vi "Main.vi"(11 "Module Admin":refnum<class "Delacor_lib_QMH_Module Admin.lvclass">) -> ()   [LabVIEW 2019, in "Calculadora.lvlib"]
doc: "This template is based off of the Queued Message Handler design pattern and the Queued Message Handler project template that ships with LabVIEW.\n\nThe main difference is that the queue is private to this module and communication between modules is performed via Broadcast and Request events.\n\nRequest events are wrapped in public API methods and are handled in the Event Handling Loop (EHL) of this VI. Any module can register for Broadcast events sent by this module. The EHL generates messages based on user interface actions.\n\nThe Message Handling Loop (MHL) processes messages generated by the EHL, or by other messages. The messages are string values, so new messages can be added easily to the Message Cases case structure in the MHL. Each message cluster can also provide an optional value for Message Data, which is a variant that can be converted to whatever message-specific data is required.\n_____\nBased on DQMH Project Template 6.1.0.94."
uses:
  Calculadora.lvlib
  <vilib>/Delacor/Delacor QMH/Libraries/Module Admin_class/Delacor_lib_QMH_Module Admin.lvclass
  Module Data--cluster.ctl
  Do Something Argument--cluster.ctl
  <vilib>/Delacor/Delacor QMH/Libraries/Message Queue_class/Delacor_lib_QMH_Message Queue.lvclass/Delacor_lib_QMH_Message Queue.ctl
  Do Something Else Argument--cluster.ctl
  Do Something Else and Wait for Reply Argument--cluster.ctl
  Do Something Else and Wait (Reply Payload)--cluster.ctl
  Stop Argument--cluster.ctl
  <vilib>/Delacor/Delacor QMH/Libraries/Module Admin_class/Delacor_lib_QMH_Module Admin.lvclass/Delacor_lib_QMH_Module Admin.ctl
  Suma Argument--cluster.ctl
  Resta Argument--cluster.ctl
  Multiplicacion Argument--cluster.ctl
  Division Argument--cluster.ctl
  Borrar Argument--cluster.ctl
  <vilib>/Utility/miscctls.llb/LVPointTypeDef.ctl
  <vilib>/Delacor/Delacor QMH/Libraries/Message Queue_class/Delacor_lib_QMH_Enqueue Message (Single).vi
  <vilib>/Delacor/Delacor QMH/Libraries/Module Admin_class/Delacor_lib_QMH_Get External Launch.vi
  <vilib>/Utility/error.llb/Error Cluster From Error Code.vi
  <vilib>/ErrorRing/Error Ring.xnode
  <vilib>/Delacor/Delacor QMH/Libraries/Message Queue_class/Delacor_lib_QMH_Message Queue.lvclass
panel:
  out "error out":errorcluster
  out "X":dbl
  out "Status":string
  in  "Simulate MHL Error":bool
  in  "Simulate EHL Error":bool
  in  "Do Something Else <Replace Me>":bool
  in  "Do Something <Replace Me>":bool
  # "These controls have associated \"Value Changed\" events configured in the Event Structure on the diagram.\n\nReplace them (and reconfigure the Event Structure) with the controls you need for your application. \n\nOther QMH Modules communicate with this Module via its Public API (wrappers for its Request Events).\n\nThis Module communicates with other Modules via its Broadcast Events.\nAny module that wants to get these messages, just registers for this module's Broadcast events."
  # "This template is for the Delacor Modified Queued Message Handler design pattern.\n\nSee the block diagram for more information on how to use this template."
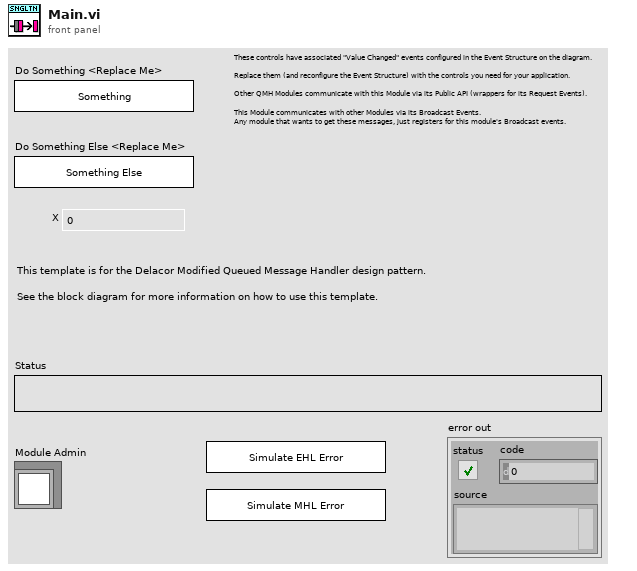
[diagram p1: front panel]
types:
  T1 = typedef "Calculadora.lvlib/Request Events--cluster.ctl" = cluster{"Stop Module":refnum<user-event>, "Do Something":refnum<user-event>, "Do Something Else":refnum<user-event>, "Do Something Else and Wait for Reply":refnum<user-event>, "Show Panel":refnum<user-event>, "Hide Panel":refnum<user-event>, "Get Module Execution Status":refnum<user-event>, "Show Diagram":refnum<user-event>, "Suma":refnum<user-event>, "Resta":refnum<user-event>, "Multiplicacion":refnum<user-event>, "Division":refnum<user-event>, "Borrar":refnum<user-event>}
  T2 = typedef "Calculadora.lvlib/Module Data--cluster.ctl" = cluster{"Status":string, "Resultado":dbl}
  T3 = typedef "Calculadora.lvlib/Do Something Argument--cluster.ctl" = cluster{"Do Something Msg":string}
  T4 = typedef "Calculadora.lvlib/Do Something Else Argument--cluster.ctl" = cluster{"Do Something Else Msg":string, "X":dbl}
  T5 = typedef "Calculadora.lvlib/Do Something Else and Wait for Reply Argument--cluster.ctl" = cluster{"Do Something Else Msg":string, "X":dbl, "Wait Notifier":refnum<notifier>, "wait for reply":bool}
  T6 = enum32{"invalid lock state", "Not Locked", "Locked (No Password)", "Password-protected"}
  T7 = typedef "Calculadora.lvlib/Stop Argument--cluster.ctl" = cluster{"Origin":string, "Exit via Stop Module Req?":bool, "Wait for Module to stop?":bool}
  T8 = typedef "Calculadora.lvlib/Suma Argument--cluster.ctl" = cluster{"Numero":dbl}
  T9 = typedef "Calculadora.lvlib/Resta Argument--cluster.ctl" = cluster{"Numero":dbl}
  T10 = typedef "Calculadora.lvlib/Multiplicacion Argument--cluster.ctl" = cluster{"Numero":dbl}
  T11 = typedef "Calculadora.lvlib/Division Argument--cluster.ctl" = cluster{"Numero":dbl}
  T12 = typedef "Calculadora.lvlib/Borrar Argument--cluster.ctl" = cluster{"Boolean":bool}
  T13 = typedef "LVPointTypeDef.ctl" = cluster{"Horizontal":i16, "Vertical":i16}
  T14 = enum32{"Invalid", "Standard", "Closed", "Hidden", "Minimized", "Maximized"}
  T15 = typedef "Calculadora.lvlib/Do Something Else and Wait (Reply Payload)--cluster.ctl" = cluster{"Value":dbl, "error":errorcluster}
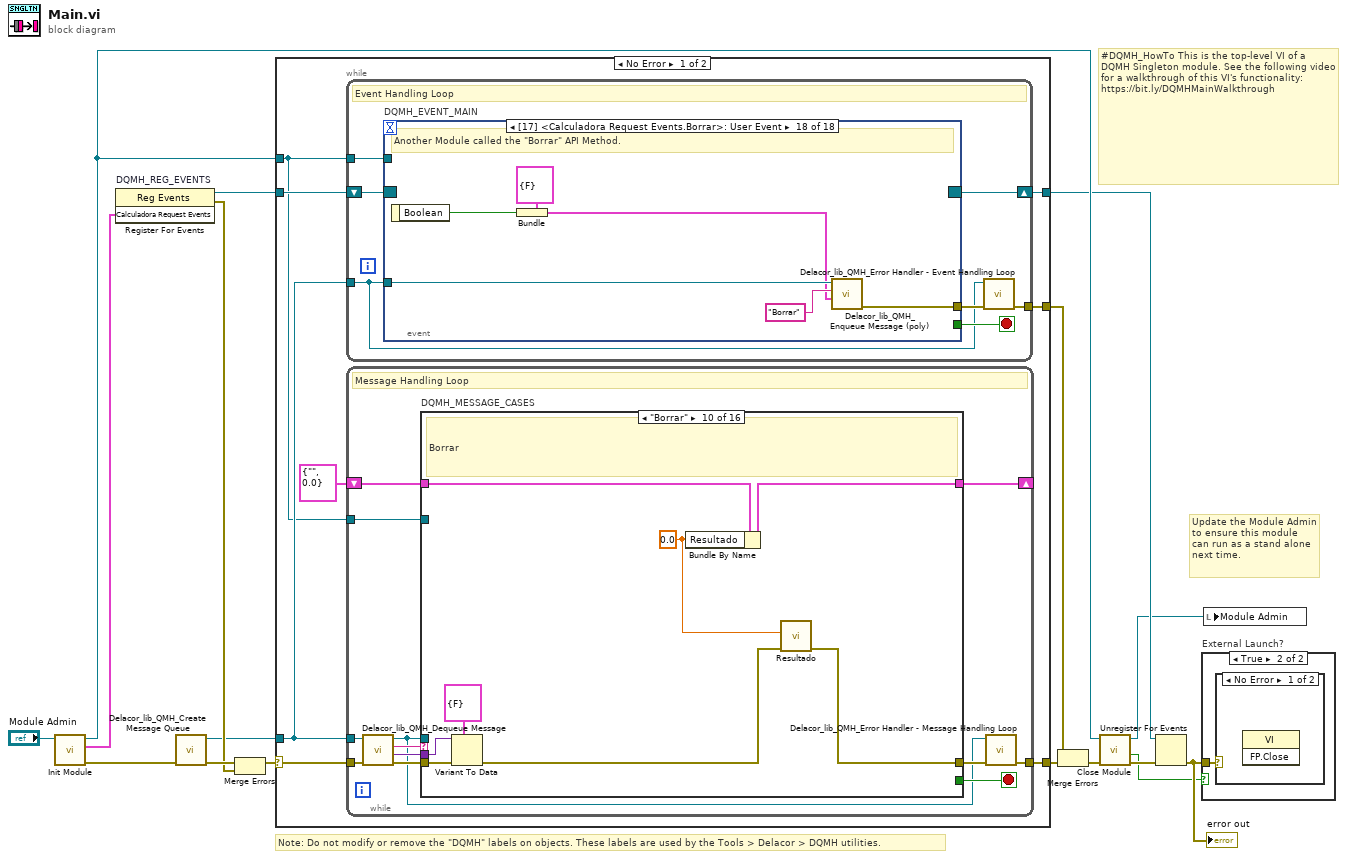
[diagram p0: block diagram]
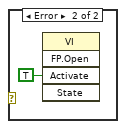
[diagram p3: hidden frame]
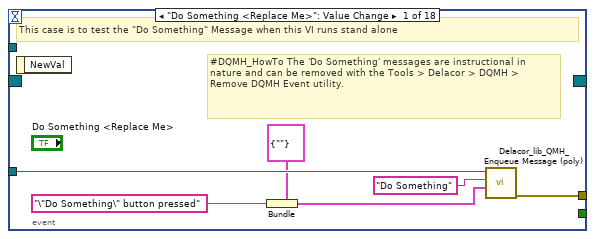
[diagram p4: hidden frame]
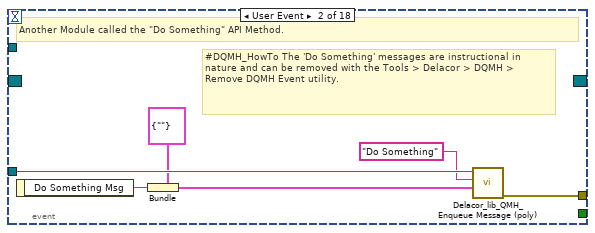
[diagram p5: hidden frame]
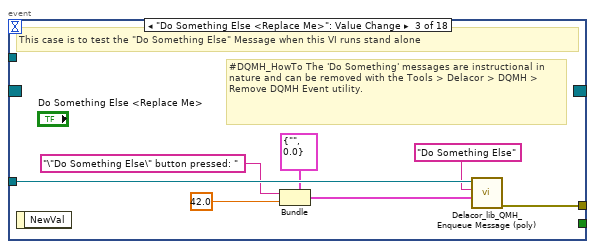
[diagram p6: hidden frame]
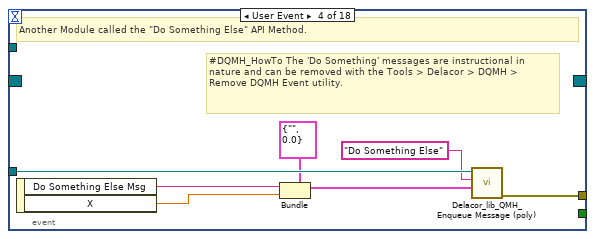
[diagram p7: hidden frame]
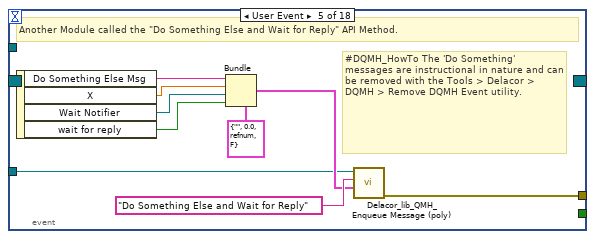
[diagram p8: hidden frame]
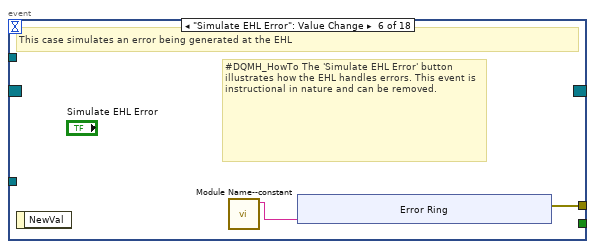
[diagram p9: hidden frame]
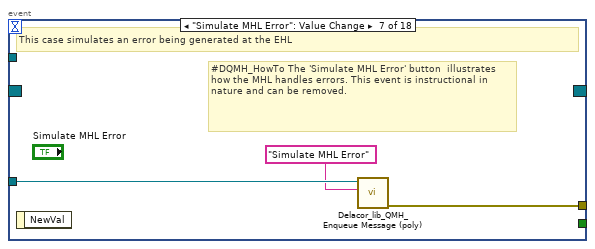
[diagram p10: hidden frame]
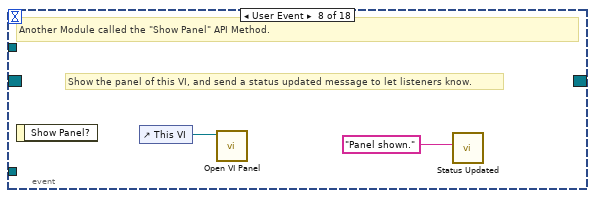
[diagram p11: hidden frame]
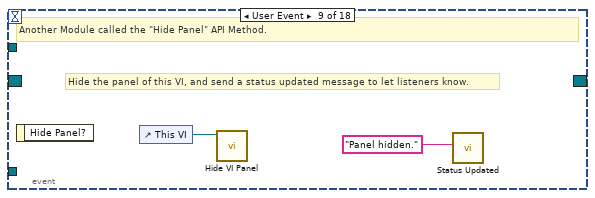
[diagram p12: hidden frame]
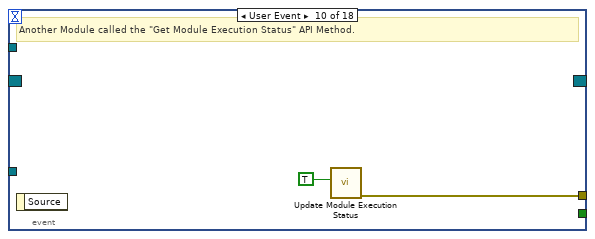
[diagram p13: hidden frame]
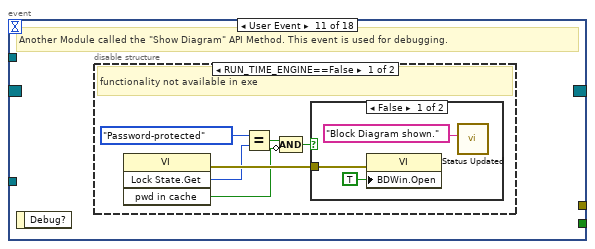
[diagram p14: hidden frame]
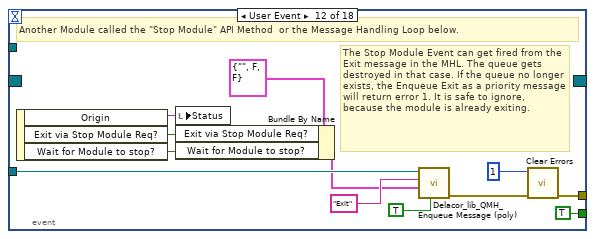
[diagram p17: hidden frame]
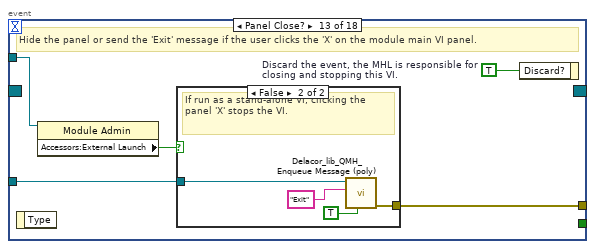
[diagram p18: hidden frame]
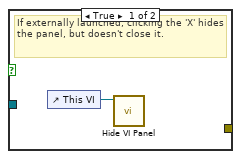
[diagram p19: hidden frame]
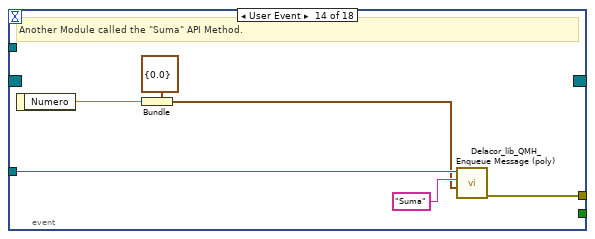
[diagram p20: hidden frame]
diagram:
  # "#DQMH_HowTo This is the top-level VI of a DQMH Singleton module. See the following video for a walkthrough of this VI's functionality: https://bit.ly/DQMHMainWalkthrough"
  # "Note: Do not modify or remove the \"DQMH\" labels on objects. These labels are used by the Tools > Delacor > DQMH utilities."
  # "Update the Module Admin to ensure this module can run as a stand alone next time."
  n1 = call "Init Module.vi"("Singleton Module Admin in"="Module Admin") -> ("error out"=w16:errorcluster, "Calculadora Request Events"=w5:T1, "Singleton Module Admin out"=w8:refnum<class "Delacor_lib_QMH_Module Admin.lvclass">)  [unwired: 8 in]
  n2 = register-events "DQMH_REG_EVENTS"(w5) -> (reference out=w6:refnum<event-registration>, error out=w9:errorcluster)  [unwired: 2 in]
  n3 = call <vilib>:"Delacor_lib_QMH_Create Message Queue.vi"("error in"=w16) -> ("error out"=w11:errorcluster, "Message Queue"=w4:refnum<class "Delacor_lib_QMH_Message Queue.lvclass">)  [unwired: 9 in]
  n4 = Merge Errors(w11, w9) -> (w10:errorcluster)
  n5 = case shown="No Error" w10 {
    selector: w10 -> [w23 w345]
    tunnel: [w25 w344] -> w17
    tunnel: [w22 w350] -> w7
    tunnel: w6 -> [w20 w350]
    tunnel: w4 -> [w19 w343]
    tunnel: [w24 _] -> w14
    tunnel: w8 -> [w18 w346]
    frame No Error {
      n6 = while {
        tunnel: w19 -> [w26]
        shift-right: [w29] -> w22
        shift-left: w20 -> [w30]
        tunnel: [w31] -> w24
        tunnel: w18 -> [w27]
        stop <- w28 stop-if-true
        # "Event Handling Loop"
        n7 = event "DQMH_EVENT_MAIN" shown="[17] <Calculadora Request Events.Borrar>: User Event" {
          selector: w30 -> [_ _ _ _ _ _ _ _ _ _ _ _ _ _ _ _ _ _]
          dyn-events: [_ _ _ _ _ _ _ _ _ _ _ _ _ _ _ _ _ _] -> w29
          timeout: _ -> [_ _ _ _ _ _ _ _ _ _ _ _ _ _ _ _ _ _]
          tunnel: [_ _ _ _ _ _ _ _ _ _ _ TRUE ("Discard?") _ _ _ _ _ _] -> w28
          tunnel: w26 -> [w37 w43 w50 w57 w60 _ w78 _ _ _ _ w102 w109 w122 w128 w134 w140 w146]
          tunnel: [w38 w44 w51 w58 w67 w69 w79 _ _ w85 _ w105 w111 w117 w123 w129 w135 w141] -> w32
          tunnel: w27 -> [_ _ _ _ _ _ _ _ _ _ _ _ w108 _ _ _ _ _]
          event "Do Something <Replace Me>": Value Change {
            # "#DQMH_HowTo The 'Do Something' messages are instructional in nature and can be removed with the Tools > Delacor > DQMH > Remove DQMH Event utility."
            # "This case is to test the \"Do Something\" Message when this VI runs stand alone"
            n8 = event-data() -> ()  [unwired: 1 in, 1 out]
            n9 = Bundle(cluster=T3 {"Do Something Msg"=""} ("Do Something Argument"), "Do Something Msg"="\"Do Something\" button pressed" ("\"Do Something\" button pressed")) -> (w33:T3)
            n10 = call-poly <vilib>:"Delacor_lib_QMH_Enqueue Message (poly).vi"("Message Data"=w33, "Message"="Do Something", "Message Queue in"=w37) -> ("error out"=w38:errorcluster)  [unwired: 7 in, 1 out]
          }
          event User Event {
            # "#DQMH_HowTo The 'Do Something' messages are instructional in nature and can be removed with the Tools > Delacor > DQMH > Remove DQMH Event utility."
            # "Another Module called the \"Do Something\" API Method."
            n11 = event-data() -> ("Do Something Msg"=w40:string)  [unwired: 1 in]
            n12 = Bundle(cluster=T3 {"Do Something Msg"=""} ("Do Something Argument"), "Do Something Msg"=w40) -> (w39:T3)
            n13 = call-poly <vilib>:"Delacor_lib_QMH_Enqueue Message (poly).vi"("Message Data"=w39, "Message"="Do Something", "Message Queue in"=w43) -> ("error out"=w44:errorcluster)  [unwired: 7 in, 1 out]
          }
          event "Do Something Else <Replace Me>": Value Change {
            # "#DQMH_HowTo The 'Do Something' messages are instructional in nature and can be removed with the Tools > Delacor > DQMH > Remove DQMH Event utility."
            # "This case is to test the \"Do Something Else\" Message when this VI runs stand alone"
            n14 = event-data() -> ()  [unwired: 1 in, 1 out]
            n15 = Bundle(cluster=T4 {"Do Something Else Msg"="", "X"=0.0} ("Do Something Else Argument"), "Do Something Else Msg"="\"Do Something Else\" button pressed: " ("\"Do Something Else\" button pressed"), "X"=42.0) -> (w47:T4)
            n16 = call-poly <vilib>:"Delacor_lib_QMH_Enqueue Message (poly).vi"("Message Data"=w47, "Message"="Do Something Else", "Message Queue in"=w50) -> ("error out"=w51:errorcluster)  [unwired: 7 in, 1 out]
          }
          event User Event {
            # "#DQMH_HowTo The 'Do Something' messages are instructional in nature and can be removed with the Tools > Delacor > DQMH > Remove DQMH Event utility."
            # "Another Module called the \"Do Something Else\" API Method."
            n17 = event-data() -> ("Do Something Else Msg"=w53:string, "X"=w52:dbl)  [unwired: 1 in]
            n18 = Bundle(cluster=T4 {"Do Something Else Msg"="", "X"=0.0} ("Do Something Else Argument"), "Do Something Else Msg"=w53, "X"=w52) -> (w54:T4)
            n19 = call-poly <vilib>:"Delacor_lib_QMH_Enqueue Message (poly).vi"("Message Data"=w54, "Message"="Do Something Else", "Message Queue in"=w57) -> ("error out"=w58:errorcluster)  [unwired: 7 in, 1 out]
          }
          event User Event {
            # "#DQMH_HowTo The 'Do Something' messages are instructional in nature and can be removed with the Tools > Delacor > DQMH > Remove DQMH Event utility."
            # "Another Module called the \"Do Something Else and Wait for Reply\" API Method."
            n20 = event-data() -> ("Do Something Else Msg"=w63:string, "X"=w62:dbl, "Wait Notifier"=w61:refnum<notifier>, "wait for reply"=w59:bool)  [unwired: 1 in]
            n21 = Bundle(cluster=T5 {"Do Something Else Msg"="", "X"=0.0, "Wait Notifier"=refnum, "wait for reply"=FALSE} ("Do Something Else and Wait for Reply Argument"), "Do Something Else Msg"=w63, "X"=w62, "Wait Notifier"=w61, "wait for reply"=w59) -> (w64:T5)
            n22 = call-poly <vilib>:"Delacor_lib_QMH_Enqueue Message (poly).vi"("Message Data"=w64, "Message"="Do Something Else and Wait for Reply", "Message Queue in"=w60) -> ("error out"=w67:errorcluster)  [unwired: 7 in, 1 out]
          }
          event "Simulate EHL Error": Value Change {
            # "#DQMH_HowTo The 'Simulate EHL Error' button  illustrates how the EHL handles errors. This event is instructional in nature and can be removed."
            # "This case simulates an error being generated at the EHL"
            n23 = event-data() -> ()  [unwired: 1 in, 1 out]
            n24 = call "Module Name--constant.vi"() -> ("Module Name"=w68:string)  [unwired: 11 in]
            n25 = xnode "Error Ring"("parameter 0"=w68) -> ("error out"=w69:errorcluster)
          }
          event "Simulate MHL Error": Value Change {
            # "#DQMH_HowTo The 'Simulate MHL Error' button  illustrates how the MHL handles errors. This event is instructional in nature and can be removed."
            # "This case simulates an error being generated at the EHL"
            n26 = event-data() -> ()  [unwired: 1 in, 1 out]
            n27 = call-poly <vilib>:"Delacor_lib_QMH_Enqueue Message (poly).vi"("Message"="Simulate MHL Error", "Message Queue in"=w78) -> ("error out"=w79:errorcluster)  [unwired: 8 in, 1 out]
          }
          event User Event {
            # "Show the panel of this VI, and send a status updated message to let listeners know."
            # "Another Module called the \"Show Panel\" API Method."
            n28 = event-data() -> ()  [unwired: 1 in, 1 out]
            n29 = control-ref of="This VI"() -> (w81:refnum<vi>)
            n30 = call "Open VI Panel.vi"("VI"=w81) -> ()  [unwired: 10 in, 1 out]
            n31 = call "Status Updated.vi"("Status"="Panel shown." ("format string")) -> ()  [unwired: 10 in, 1 out]
          }
          event User Event {
            # "Hide the panel of this VI, and send a status updated message to let listeners know."
            # "Another Module called the \"Hide Panel\" API Method."
            n32 = event-data() -> ()  [unwired: 1 in, 1 out]
            n33 = control-ref of="This VI"() -> (w83:refnum<vi>)
            n34 = call "Hide VI Panel.vi"("VI"=w83) -> ()  [unwired: 10 in, 1 out]
            n35 = call "Status Updated.vi"("Status"="Panel hidden." ("format string")) -> ()  [unwired: 10 in, 1 out]
          }
          event User Event {
            # "Another Module called the \"Get Module Execution Status\" API Method."
            n36 = event-data() -> ()  [unwired: 1 in, 1 out]
            n37 = call "Update Module Execution Status.vi"("Running?"=TRUE) -> ("error out"=w85:errorcluster)  [unwired: 10 in]
          }
          event User Event {
            # "Another Module called the \"Show Diagram\" API Method. This event is used for debugging."
            n38 = event-data() -> ()  [unwired: 1 in, 1 out]
            n39 = disable-structure shown="RUN_TIME_ENGINE==False" {
              frame condition #0 (active) {
                # "functionality not available in exe"
                n40 = invoke class="VI" method="Lock State.Get"() -> (error out=w91:errorcluster, "Get Lock State"=w90:T6, "pwd in cache"=w87:bool)  [unwired: 4 in, 1 out]
                n41 = Equal?(x=T6."Password-protected", y=w90) -> (x = y?=w88:bool)
                n42 = Compound Arithmetic op=AND(w88, invert w87) -> (w86:bool)
                n43 = case shown="False" w86 {
                  tunnel: w91 -> [w94 _]
                  frame False {
                    n44 = property class="VI"(error in=w94, "BDWin.Open"=TRUE ("Block Diagram Window:Open")) -> ()  [unwired: 1 in, 2 out]
                    n45 = call "Status Updated.vi"("Status"="Block Diagram shown." ("format string")) -> ()  [unwired: 10 in, 1 out]
                  }
                  frame True {
                    # "Password-protected VI, and the password is not in the cache. Do not show the diagram."
                  }
                }
              }
              frame condition #1 {
              }
            }
          }
          event User Event {
            # "The Stop Module Event can get fired from the Exit message in the MHL. The queue gets destroyed in that case. If the queue no longer exists, the Enqueue Exit as a priority message will return error 1. It is safe to ignore, because the module is already exiting."
            # "Another Module called the \"Stop Module\" API Method  or the Message Handling Loop below."
            n46 = event-data() -> ("Origin"=w101:string, "Exit via Stop Module Req?"=w97:bool, "Wait for Module to stop?"=w96:bool)  [unwired: 1 in]
            n47 = local write "Status"(w101) -> ()
            n48 = Bundle By Name(cluster=T7 {"Origin"="", "Exit via Stop Module Req?"=FALSE, "Wait for Module to stop?"=FALSE} ("Stop Argument"), "Exit via Stop Module Req?"=w97, "Wait for Module to stop?"=w96) -> (w95:T7)
            n49 = call-poly <vilib>:"Delacor_lib_QMH_Enqueue Message (poly).vi"("Priority Message? (F)"=TRUE, "Message Data"=w95, "Message"="Exit", "Message Queue in"=w102) -> ("error out"=w106:errorcluster)  [unwired: 6 in, 1 out]
            n50 = call <vilib>:"Clear Errors.vi"("error in (no error)"=w106, "specific error code to clear (0: all)"=1) -> ("error out"=w105:errorcluster)  [unwired: 4 in, 1 out]
          }
          event Panel Close? {
            w110 = TRUE  # Discard the event, the MHL is responsible for closing and stopping this VI.
            # "Hide the panel or send the 'Exit' message if the user clicks the 'X' on the module main VI panel."
            n51 = event-data() -> ()  [unwired: 1 in, 1 out]
            n52 = property class="Module Admin"(reference=w108) -> ("Accessors:External Launch"=w107:bool)  [unwired: 1 in, 2 out]
            n53 = case shown="False" w107 {
              tunnel: w109 -> [_ w115]
              tunnel: [_ w116] -> w111
              frame True {
                # "If externally launched, clicking the 'X' hides the panel, but doesn't close it."
                n54 = control-ref of="This VI"() -> (w112:refnum<vi>)
                n55 = call "Hide VI Panel.vi"("VI"=w112) -> ()  [unwired: 10 in, 1 out]
              }
              frame False {
                # "If run as a stand-alone VI, clicking the panel 'X' stops the VI."
                n56 = call-poly <vilib>:"Delacor_lib_QMH_Enqueue Message (poly).vi"("Priority Message? (F)"=TRUE, "Message"="Exit", "Message Queue in"=w115) -> ("error out"=w116:errorcluster)  [unwired: 7 in, 1 out]
              }
            }
            n57 = event-data("Discard?"=w110) -> ()  [unwired: 1 in, 1 out]
          }
          event User Event {
            # "Another Module called the \"Suma\" API Method."
            n58 = event-data() -> ("Numero"=w118:dbl)  [unwired: 1 in]
            n59 = Bundle(cluster=T8 {"Numero"=0.0} ("Suma Argument"), "Numero"=w118) -> (w119:T8)
            n60 = call-poly <vilib>:"Delacor_lib_QMH_Enqueue Message (poly).vi"("Message Data"=w119, "Message"="Suma", "Message Queue in"=w122) -> ("error out"=w117:errorcluster)  [unwired: 7 in, 1 out]
          }
          event User Event {
            # "Another Module called the \"Resta\" API Method."
            n61 = event-data() -> ("Numero"=w124:dbl)  [unwired: 1 in]
            n62 = Bundle(cluster=T9 {"Numero"=0.0} ("Resta Argument"), "Numero"=w124) -> (w125:T9)
            n63 = call-poly <vilib>:"Delacor_lib_QMH_Enqueue Message (poly).vi"("Message Data"=w125, "Message"="Resta", "Message Queue in"=w128) -> ("error out"=w123:errorcluster)  [unwired: 7 in, 1 out]
          }
          event User Event {
            # "Another Module called the \"Multiplicacion\" API Method."
            n64 = event-data() -> ("Numero"=w130:dbl)  [unwired: 1 in]
            n65 = Bundle(cluster=T10 {"Numero"=0.0} ("Multiplicacion Argument"), "Numero"=w130) -> (w131:T10)
            n66 = call-poly <vilib>:"Delacor_lib_QMH_Enqueue Message (poly).vi"("Message Data"=w131, "Message"="Multiplicacion", "Message Queue in"=w134) -> ("error out"=w129:errorcluster)  [unwired: 7 in, 1 out]
          }
          event User Event {
            # "Another Module called the \"Division\" API Method."
            n67 = event-data() -> ("Numero"=w136:dbl)  [unwired: 1 in]
            n68 = Bundle(cluster=T11 {"Numero"=0.0} ("Division Argument"), "Numero"=w136) -> (w137:T11)
            n69 = call-poly <vilib>:"Delacor_lib_QMH_Enqueue Message (poly).vi"("Message Data"=w137, "Message"="Division", "Message Queue in"=w140) -> ("error out"=w135:errorcluster)  [unwired: 7 in, 1 out]
          }
          event User Event {
            # "Another Module called the \"Borrar\" API Method."
            n70 = event-data() -> ("Boolean"=w142:bool)  [unwired: 1 in]
            n71 = Bundle(cluster=T12 {"Boolean"=FALSE} ("Borrar Argument"), "Boolean"=w142) -> (w143:T12)
            n72 = call-poly <vilib>:"Delacor_lib_QMH_Enqueue Message (poly).vi"("Message Data"=w143, "Message"="Borrar", "Message Queue in"=w146) -> ("error out"=w141:errorcluster)  [unwired: 7 in, 1 out]
          }
        }
        n73 = call-dynamic "Delacor_lib_QMH_Error Handler - Event Handling Loop.vi"("error in"=w32, "Message Queue in"=w26) -> ("dup error in"=w31:errorcluster)  [unwired: 8 in, 1 out]
      }
      n74 = while {
        tunnel: w19 -> [w149]
        shift-right: [w153] -> _
        shift-left: T2 {"Status"="", "Resultado"=0.0} ("Data Cluster") -> [w154]
        tunnel: w23 -> [w157]
        tunnel: [w155] -> w25
        tunnel: w18 -> [w147]
        stop <- w152 stop-if-true
        # "Message Handling Loop"
        n75 = call-dynamic "Delacor_lib_QMH_Dequeue Message.vi"("error in"=w157, "Message Queue in"=w149) -> ("error out"=w156:errorcluster, "Message Data"=w150:variant, "Message"=w151:string, "Message Queue out"=w148:refnum<class "Delacor_lib_QMH_Message Queue.lvclass">)  [unwired: 6 in]
        n76 = case "DQMH_MESSAGE_CASES" shown="\"Borrar\"" w151 {
          selector: w151 -> [_ _ _ _ _ _ _ _ _ _ _ _ _ _ _ w330]
          tunnel: w148 -> [_ _ _ _ _ _ _ _ _ _ _ _ _ w300 w322 _]
          tunnel: w156 -> [w177 w181 w189 w198 w217 w240 w250 w261 w272 w280 w283 w285 w290 w307 w328 w332]
          tunnel: [w175 w181 w187 w197 w216 w230 w249 w251 w262 w273 w282 w285 w289 w303 w325 w333] -> w158
          tunnel: w154 -> [w166 w180 w186 w196 w214 w236 w242 w254 w265 w279 w281 w284 w287 w302 w321 w331]
          tunnel: [w165 w180 w186 w196 w214 w233 w241 w253 w264 w276 w281 w284 w287 w302 w321 w331] -> w153
          tunnel: [_ _ _ _ _ _ _ _ _ _ _ _ _ _ w320 _] -> w152
          tunnel: w150 -> [_ _ w185 w193 w211 w239 w248 w260 w271 w278 _ _ _ w301 w319 _]
          tunnel: w147 -> [w167 _ _ _ _ _ _ _ _ _ _ _ _ w299 w314 _]
          frame "Initialize" {
            w161 = "Initial Message" ("Initial Message")
            # "Initialize - Any operation that needs to be done before the module can receive messages. Synchronize Caller Events.vi will inform Start Module.vi that the module has launched and is ready to receive messages. Module Did Init.vi will broadcast that the module initialized."
            n77 = call "Synchronize Caller Events.vi"("error in (no error)"=w177, "Singleton Module Admin in"=w167) -> ("error out"=w176:errorcluster, "Singleton Module Admin out"=w162:refnum<class "Delacor_lib_QMH_Module Admin.lvclass">)  [unwired: 8 in]
            n78 = property class="Module Admin"(reference=w162) -> ("Accessors:External Launch"=w171:bool)  [unwired: 1 in, 2 out]
            n79 = Select(t=T14."Hidden" ("State"), s=w171, f=T14."Standard" ("State")) -> (s? t:f=w168:T14)
            n80 = call "Module Name--constant.vi"() -> ("Module Name"=w174:string)  [unwired: 11 in]
            n81 = property class="VI"("Front Panel.Title"=w174) -> (reference out=w173:refnum<vi>, error out=w179:errorcluster)  [unwired: 2 in]
            n82 = call "Module Name--constant.vi"() -> ("Module Name"=w163:string)  [unwired: 11 in]
            n83 = invoke class="VI" method="FP.Open"(reference=w173, error in=w179, "State"=w168) -> (reference out=w172:refnum<vi>, error out=w178:errorcluster)  [unwired: 2 in, 3 out]
            n84 = Bundle By Name(cluster=w166, "Resultado"=0.0, "Status"=w161) -> (w165:T2)
            n85 = call "Module Did Init.vi"("error in (no error)"=w176, "Initialized?"=TRUE, "Origin"=w163) -> ("error out"=w175:errorcluster)  [unwired: 8 in]
            n86 = invoke class="VI" method="FP.Center"(reference=w172, error in=w178) -> ()  [unwired: 1 in, 3 out]
            n87 = property on="Pane" class="Pane"("Origin"=T13 {"Horizontal"=0, "Vertical"=0}) -> ()  [unwired: 2 in, 2 out]
            "Status" <- w161
          }
          frame "---Module Specific---" {
            # "Separator -- The following cases handle messages specific to this Module."
          }
          frame "Do Something" {
            # "#DQMH_HowTo The 'Do Something' messages are instructional in nature and can be removed with the Tools > Delacor > DQMH > Remove DQMH Event utility."
            # "Do Something - Replace this message with functionality for your own application. Note that this message also fires the \"Did Something\" broadcast event."
            n88 = Variant To Data(error in=w189, type=T3 {"Do Something Msg"=""} ("Do Something Argument"), Variant=w185) -> (data=w184:T3, error out=w188:errorcluster)
            n89 = Unbundle By Name(w184) -> ("Do Something Msg"=w182:string)
            n90 = call "Did Something.vi"("error in (no error)"=w188, "Did Something Msg"=w182) -> ("error out"=w187:errorcluster)  [unwired: 9 in]
            n91 = local write "Status"(w182) -> ()
            n92 = call "Status Updated.vi"("Status"=w182) -> ()  [unwired: 10 in, 1 out]
          }
          frame "Do Something Else" {
            # "#DQMH_HowTo The 'Do Something' messages are instructional in nature and can be removed with the Tools > Delacor > DQMH > Remove DQMH Event utility."
            # "Do Something Else - Replace this message with functionality for your own application."
            n93 = Variant To Data(error in=w198, type=T4 {"Do Something Else Msg"="", "X"=0.0} ("Do Something Else Argument"), Variant=w193) -> (data=w194:T4, error out=w197:errorcluster)
            n94 = Unbundle By Name(w194) -> ("Do Something Else Msg"=w192:string, "X"=w191:dbl)
            "X" <- w191
            n95 = Format Into String(initial string=w192, w191) -> (resulting string=w190:string)  [unwired: 2 in, 1 out]
            n96 = local write "Status"(w190) -> ()
            n97 = call "Status Updated.vi"("Status"=w190) -> ()  [unwired: 10 in, 1 out]
          }
          frame "Do Something Else and Wait for Reply" {
            w206 = "X(%.2f)+Offset(%.2f)=%.2f"  # status message format string
            # "#DQMH_HowTo The 'Do Something' messages are instructional in nature and can be removed."
            # "Send back X with a random offset"
            # "Do Something Else and Wait for Reply - Replace this message with functionality for your own application. Note that this message must fire a notifier to let callers know it has finished execution, and it returns an error if the 'Value' is negative."
            n98 = Random Number (0-1)() -> (number: 0 to 1=w208:dbl)
            n99 = Variant To Data(error in=w217, type=T5 {"Do Something Else Msg"="", "X"=0.0, "Wait Notifier"=refnum, "wait for reply"=FALSE} ("Do Something Else and Wait for Reply Argument"), Variant=w211) -> (data=w212:T5, error out=w215:errorcluster)
            n100 = Unbundle By Name(w212) -> ("Wait Notifier"=w199:refnum<notifier>, "Do Something Else Msg"=w210:string, "X"=w207:dbl, "wait for reply"=w203:bool)
            n101 = Add(x=w208, y=w207) -> (x+y=w202:dbl)
            n102 = local write "X"(w207) -> ()
            n103 = Less Than 0?(x=w202) -> (x < 0?=w205:bool)
            n104 = Format Into String(format string=w206, initial string=w210, w207, w208, w202) -> (resulting string=w204:string)  [unwired: 1 in, 1 out]
            n105 = case shown="True" w205 {
              tunnel: [_ w224] -> w200
              frame False {
              }
              frame True {
                n106 = xnode "Error Ring"() -> ("error out"=w224:errorcluster)
              }
            }
            n107 = Bundle By Name(cluster=T15 {"Value"=0.0, "error"={"status"=FALSE, "code"=0, "source"=""}} ("notification"), "error"=w200, "Value"=w202) -> (w201:T15)
            n108 = local write "Status"(w204) -> ()
            n109 = call "Status Updated.vi"("Status"=w204) -> ()  [unwired: 10 in, 1 out]
            n110 = case shown="True" w203 {
              tunnel: w201 -> [_ w220]
              tunnel: w199 -> [_ w219]
              frame False {
              }
              frame True {
                # "Simulate an operation that requires a wait."
                n111 = flat-sequence {
                  tunnel: w220 -> [w223]
                  tunnel: w219 -> [w222]
                  tunnel: w218 -> [_]
                  frame #0 {
                    n112 = Send Notification(notification=w223, notifier=w222) -> ()  [unwired: 1 in, 2 out]
                  }
                }
                n113 = Wait (ms)(milliseconds to wait=u32 1000) -> (millisecond timer value=w218:u32)
              }
            }
            n114 = Merge Errors(w215, w200) -> (w216:errorcluster)
          }
          frame "Suma" {
            # "Suma"
            n115 = Variant To Data(error in=w240, type=T8 {"Numero"=0.0} ("Suma Argument"), Variant=w239) -> (data=w237:T8, error out=w231:errorcluster)
            n116 = Unbundle By Name(w236) -> ("Resultado"=w235:dbl)
            n117 = Unbundle By Name(w237) -> ("Numero"=w234:dbl)
            n118 = Add(x=w235, y=w234) -> (x+y=w232:dbl)
            n119 = Bundle By Name(cluster=w236, "Resultado"=w232) -> (w233:T2)
            n120 = call "Resultado.vi"("error in"=w231, "Resultado"=w232) -> ("error out"=w230:errorcluster)  [unwired: 9 in]
          }
          frame "Resta" {
            # "Resta"
            n121 = Variant To Data(error in=w250, type=T9 {"Numero"=0.0} ("Resta Argument"), Variant=w248) -> (data=w243:T9, error out=w249:errorcluster)
            n122 = Unbundle By Name(w242) -> ("Resultado"=w246:dbl)
            n123 = Unbundle By Name(w243) -> ("Numero"=w245:dbl)
            n124 = Subtract(x=w246, y=w245) -> (x-y=w244:dbl)
            n125 = Bundle By Name(cluster=w242, "Resultado"=w244) -> (w241:T2)
            n126 = call "Resultado.vi"("Resultado"=w244) -> ()  [unwired: 10 in, 1 out]
          }
          frame "Multiplicacion" {
            # "Multiplicacion"
            n127 = Variant To Data(error in=w261, type=T10 {"Numero"=0.0} ("Multiplicacion Argument"), Variant=w260) -> (data=w255:T10, error out=w252:errorcluster)
            n128 = Unbundle By Name(w254) -> ("Resultado"=w258:dbl)
            n129 = Unbundle By Name(w255) -> ("Numero"=w257:dbl)
            n130 = Multiply(x=w258, y=w257) -> (x*y=w256:dbl)
            n131 = Bundle By Name(cluster=w254, "Resultado"=w256) -> (w253:T2)
            n132 = call "Resultado.vi"("error in"=w252, "Resultado"=w256) -> ("error out"=w251:errorcluster)  [unwired: 9 in]
          }
          frame "Division" {
            # "Division"
            n133 = Variant To Data(error in=w272, type=T11 {"Numero"=0.0} ("Division Argument"), Variant=w271) -> (data=w266:T11, error out=w263:errorcluster)
            n134 = Unbundle By Name(w265) -> ("Resultado"=w269:dbl)
            n135 = Unbundle By Name(w266) -> ("Numero"=w268:dbl)
            n136 = Divide(x=w269, y=w268) -> (x/y=w267:dbl)
            n137 = Bundle By Name(cluster=w265, "Resultado"=w267) -> (w264:T2)
            n138 = call "Resultado.vi"("error in"=w263, "Resultado"=w267) -> ("error out"=w262:errorcluster)  [unwired: 9 in]
          }
          frame "Borrar" {
            w275 = 0.0 ("Resultado")
            # "Borrar"
            n139 = Variant To Data(error in=w280, type=T12 {"Boolean"=FALSE} ("Borrar Argument"), Variant=w278) -> (error out=w274:errorcluster)  [unwired: 1 out]
            n140 = Bundle By Name(cluster=w279, "Resultado"=w275) -> (w276:T2)
            n141 = call "Resultado.vi"("error in"=w274, "Resultado"=w275) -> ("error out"=w273:errorcluster)  [unwired: 9 in]
          }
          frame "---Copy This Frame---" {
            # "Duplicate this frame when creating new messages.  Change this comment in the duplicated frame to describe this message."
            n142 = Merge Errors(w283) -> (w282:errorcluster)
          }
          frame "---Exit and Error Handling---" {
            # "Separator - The following cases handle errors and exit messages."
          }
          frame "Simulate MHL Error" {
            # "#DQMH_HowTo The 'Simulate MHL Error' button  illustrates how the MHL handles errors. This event is instructional in nature and can be removed."
            # "Simulate an error occurring at the MHL"
            n143 = call "Module Name--constant.vi"() -> ("Module Name"=w286:string)  [unwired: 11 in]
            n144 = xnode "Error Ring"("parameter 0"=w286) -> ("error out"=w288:errorcluster)
            n145 = Merge Errors(w290, w288) -> (w289:errorcluster)
          }
          frame "Error" {
            # "#CodeRecommended - If you ever change the name of this \"Error\" message, you'll need to update the name in the Check Loop Error.vi as well."
            # "#CodeRecommended - If the module is running in standalone mode (External Launch = FALSE), this code will pop up an error dialog and call the 'Exit' message if an error occurs. Add more fine-grained error handling here."
            # "Error - Check the error message data and respond accordingly. This message is sent by the \"Error Handler\" VIs at the end of each loop in this application."
            n146 = property class="Module Admin"(reference=w299) -> ("Accessors:External Launch"=w298:bool)  [unwired: 1 in, 2 out]
            n147 = Variant To Data(error in=w307, type=errorcluster {"status"=FALSE, "code"=0, "source"=""} ("error constant"), Variant=w301) -> (data=w308:errorcluster, error out=w305:errorcluster)
            n148 = call "Error Reported.vi"("Error"=w308) -> ()  [unwired: 10 in, 1 out]
            n149 = case shown="False" w298 {
              tunnel: [w313 _] -> w304
              tunnel: w300 -> [w311 _]
              tunnel: w308 -> [w312 _]
              frame False {
                # "If the module is running standalone, then pop up an error dialog and call the \"Exit\" message."
                n150 = call <vilib>:"Simple Error Handler.vi"("error in (no error)"=w312) -> ()  [unwired: 4 in, 5 out]
                n151 = call-poly <vilib>:"Delacor_lib_QMH_Enqueue Message (poly).vi"("Priority Message? (F)"=TRUE, "Message"="Exit", "Message Queue in"=w311) -> ("error out"=w313:errorcluster)  [unwired: 7 in, 1 out]
              }
              frame True {
                # "If the module was launched externally, calling the Error Reported broadcast VI is the only action performed by the \"Error\" message. The module's caller can then process the error appropriately."
              }
            }
            n152 = Merge Errors(w305, w304) -> (w303:errorcluster)
            n153 = local write "error out"(w303) -> ()
          }
          frame "Exit" {
            w318 = 91  # 91: not all Exit messages will have an argument
            w320 = TRUE  # Stop the VI
            # "Release the message queue reference"
            # "#CodeNeeded - Add any required cleanup code here"
            # "Exit - Exit the application."
            n154 = Variant To Data(error in=w328, type=T7 {"Origin"="", "Exit via Stop Module Req?"=FALSE, "Wait for Module to stop?"=FALSE} ("Stop Argument"), Variant=w319) -> (data=w316:T7, error out=w324:errorcluster)
            n155 = call <vilib>:"Clear Errors.vi"("error in (no error)"=w324, "specific error code to clear (0: all)"=w318) -> ("error out"=w327:errorcluster)  [unwired: 4 in, 1 out]
            n156 = control-ref of="This VI"() -> (w315:refnum<vi>)
            n157 = call-dynamic "Delacor_lib_QMH_Release Message Queue.vi"("error in"=w327, "Message Queue"=w322) -> ("error out"=w326:errorcluster)  [unwired: 9 in]
            n158 = call "Handle Exit.vi"("Stop Argument"=w316, "Admin in"=w314, "VI reference"=w315) -> ("error out"=w323:errorcluster)  [unwired: 7 in, 1 out]
            n159 = Merge Errors(w326, w323) -> (w325:errorcluster)
          }
          frame Default {
            # "'Default' case only runs if there is a message that isn't defined in any of the other cases.  Output a programming error."
            n160 = call "Module Name--constant.vi"() -> ("Module Name"=w329:string)  [unwired: 11 in]
            n161 = xnode "Error Ring"("parameter 0"=w330, "parameter 1"=w329) -> ("error out"=w334:errorcluster)
            n162 = Merge Errors(w332, w334) -> (w333:errorcluster)
          }
        }
        n163 = call-dynamic "Delacor_lib_QMH_Error Handler - Message Handling Loop.vi"("error in"=w158, "Message Queue in"=w148) -> ("dup error in"=w155:errorcluster)  [unwired: 8 in, 1 out]
      }
    }
    frame Error {
      # "Synchronize Caller Events.vi will inform Start Module.vi that the module has launched and will let the code calling Start Module.vi register for broadcasts and would permit the caller receive the broadcast that an error occurred at launch time."
      n164 = call-dynamic "Delacor_lib_QMH_Release Message Queue.vi"("error in"=w345, "Message Queue"=w343) -> ("error out"=w344:errorcluster)  [unwired: 9 in]
      n165 = call "Synchronize Caller Events.vi"("Singleton Module Admin in"=w346) -> ("error out"=w351:errorcluster)  [unwired: 9 in, 1 out]
      n166 = call "Module Name--constant.vi"() -> ("Module Name"=w349:string)  [unwired: 11 in]
      n167 = Format Into String(format string="An error occurred during initialization. %s is no longer running.", w349) -> (resulting string=w347:string)  [unwired: 2 in, 1 out]
      n168 = Merge Errors(w344, w351) -> (w352:errorcluster)
      n169 = call "Error Reported.vi"("Additional Information"=w347, "Error"=w352) -> ()  [unwired: 9 in, 1 out]
    }
  }
  n170 = Merge Errors(w14, w17) -> (w13:errorcluster)
  n171 = call "Close Module.vi"("error in (no error)"=w13, "Module Admin in"=w8) -> ("error out"=w15:errorcluster, "External Launch"=w1:bool, "Module Admin out"=w2:refnum<class "Delacor_lib_QMH_Module Admin.lvclass">)  [unwired: 7 in]
  n172 = Unregister For Events(event registration refnum=w7, error in=w15) -> (error out=w12:errorcluster)
  "error out" <- w12
  n173 = case "External Launch?" shown="True" w1 {
    tunnel: w12 -> [_ w353]
    frame False {
    }
    frame True {
      n174 = case shown="No Error" w353 {
        frame No Error {
          n175 = invoke class="VI" method="FP.Close"() -> ()  [unwired: 3 in, 3 out]
        }
        frame Error {
          n176 = invoke class="VI" method="FP.Open"("Activate"=TRUE ("Activate?")) -> ()  [unwired: 4 in, 5 out]
        }
      }
    }
  }
  n177 = local write "Module Admin"(w2) -> ()
